vi "Get Histogram data.vi"(8 "error in (no error)":errorcluster, 11 "Data In":string[][](array[string])) -> (0 "error out":errorcluster, 3 "Histogram Data":i32[](array[numeric]))   [LabVIEW 2017]
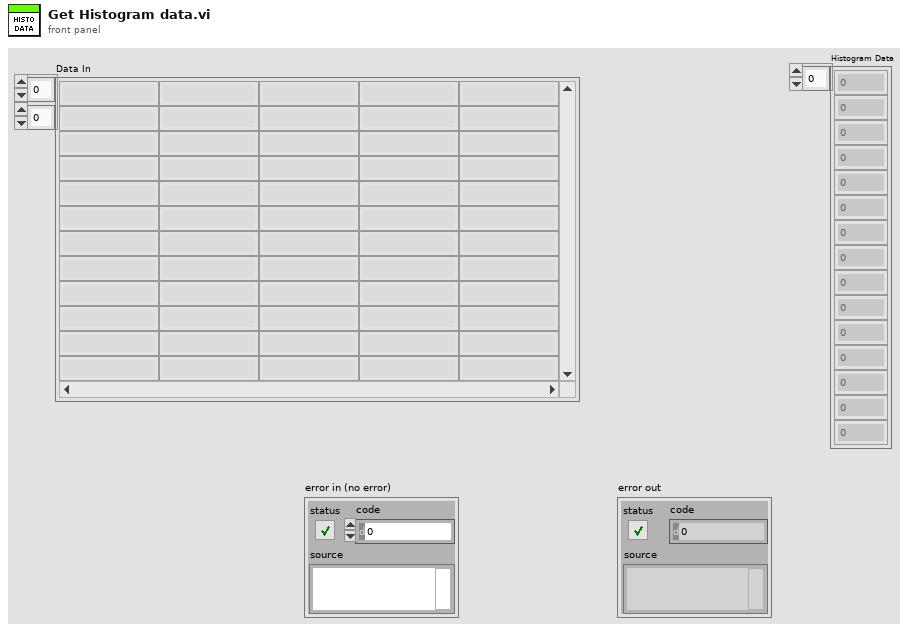
[diagram p1: front panel]
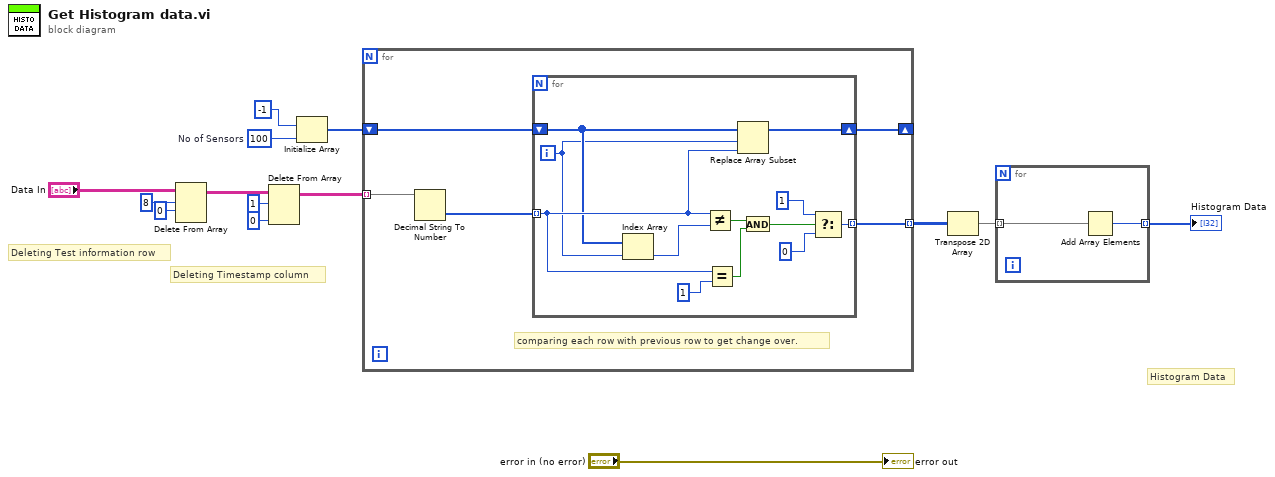
[diagram p0: block diagram]
diagram:
  w4 = 100  # No of Sensors
  # "Histogram Data"
  # "Deleting Timestamp column"
  # "Deleting Test information row"
  n1 = Delete From Array(array="Data In", length=8, index (row)=0) -> (array with subset deleted=w10:string[][])  [unwired: 1 in, 1 out]
  n2 = Delete From Array(array=w10, length=1, index (col)=0 ("disabled index (col)")) -> (array with subset deleted=w9:string[][])  [unwired: 1 in, 1 out]
  n3 = Initialize Array(-1 ("element"), w4) -> (w3:i32[])
  n4 = for {
    tunnel: w9 -> [w19] mode=indexing
    tunnel: [w17] -> w11 mode=indexing
    shift-right: [w15] -> _
    shift-left: w3 -> [w16]
    # "comparing each row with previous row to get change over."
    n5 = Decimal String To Number(string=w19) -> (number=w18:i32[])  [unwired: 2 in, 1 out]
    n6 = for {
      tunnel: w18 -> [w23] mode=indexing
      shift-right: [w31] -> w15
      shift-left: w16 -> [w22]
      tunnel: [w27] -> w17 mode=indexing
      i -> [w20]
      n7 = Index Array(array=w22, index=w20) -> (element=w21:i32)
      n8 = Not Equal?(x=w23, y=w21) -> (x != y?=w30:bool)
      n9 = Equal?(x=w23, y=1) -> (x = y?=w24:bool)
      n10 = Replace Array Subset(array=w22, new element=w23, index=w20) -> (w31:i32[])
      n11 = And(x=w30, y=w24) -> (x .and. y?=w25:bool)
      n12 = Select(t=1, s=w25, f=0) -> (s? t:f=w27:i32)
    }
  }
  n13 = Transpose 2D Array(2D array=w11) -> (transposed array=w2:i32[][])
  n14 = for {
    tunnel: [w32] -> w12 mode=indexing
    tunnel: w2 -> [w33] mode=indexing
    n15 = Add Array Elements(numeric array=w33) -> (sum=w32:i32)
  }
  "Histogram Data" <- w12
  "error out" <- "error in (no error)"
